vi "Create Event.vi"(9 "Event":refnum<class "Event.lvclass">, 10 "Self Event Alias":string, 11 "jettl Msg Create Event in":refnum<class "jettl Msg Create Event.lvclass">) -> (3 "jettl Msg Create Event out":refnum<class "jettl Msg Create Event.lvclass">)   [LabVIEW 2021, in "Create Event Msg Strategy.lvlib" / "jettl Msg Create Event.lvclass"]
uses:
  jettl Msg Create Event.lvclass
  jettl/Event/Event.lvclass
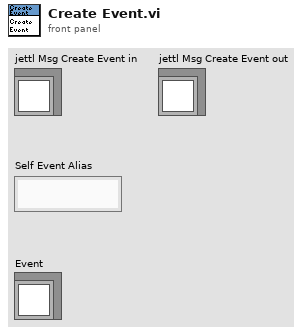
[diagram p1: front panel]
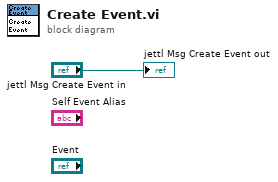
[diagram p0: block diagram]
diagram:
  "jettl Msg Create Event out" <- "jettl Msg Create Event in"
